vi "Create Table.vi"(6 "CaseSelectInput":bool, 8 "error in (no error)":errorcluster, 9 "ColumnInfo":T2[](array[typedef]), 10 "Table":string, 11 "Refnum in":T1) -> (0 "error out":errorcluster, 3 "Refnum out":T1)   [LabVIEW 2021, in "Database.lvlib"]
uses:
  Database.lvlib
  <vilib>/addons/database/Auxilliary.llb/DB Tools Column Info.ctl
  <vilib>/addons/database/Auxilliary.llb/DB Tools DataTypes.ctl
  <vilib>/addons/database/Connection.llb/Conn ObjectReference.ctl
  <vilib>/addons/database/NI_Database_API.lvlib
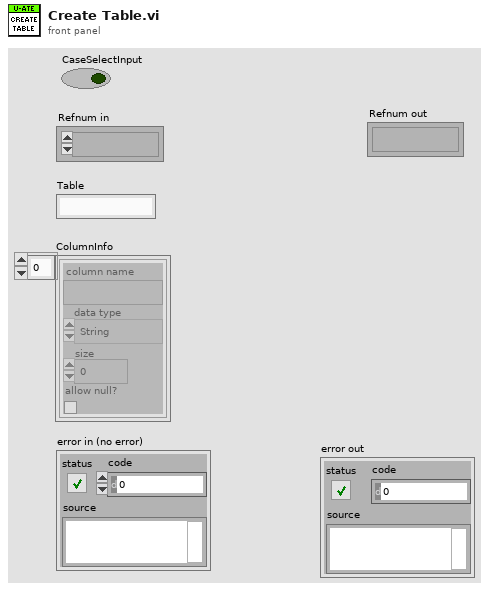
[diagram p1: front panel]
types:
  T1 = typedef "NI_Database_API.lvlib/Conn ObjectReference.ctl" = refnum<k1>
  T2 = typedef "NI_Database_API.lvlib/DB Tools Column Info.ctl" = cluster{"column name":string, "data type":T3, "size":i32, "allow null?":bool}
  T3 = typedef "NI_Database_API.lvlib/DB Tools DataTypes.ctl" = enum16{"String", "Long (I32)", "Single (SGL)", "Double (DBL)", "Date/Time", "Binary"}
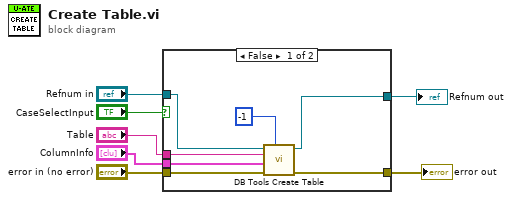
[diagram p0: block diagram]
diagram:
  n1 = case shown="False" "CaseSelectInput" {
    tunnel: "error in (no error)" -> [w13 w15]
    tunnel: "Refnum in" -> [w12 w16]
    tunnel: "Table" -> [w11 _]
    tunnel: "ColumnInfo" -> [w10 _]
    tunnel: [w9 w15] -> w4
    tunnel: [w8 w16] -> w5
    frame False {
      n2 = call <vilib>:"DB Tools Create Table.vi"("primary key (-1)"=-1, "error in (no error)"=w13, "column information"=w10, "table"=w11, "connection reference"=w12) -> ("error out"=w9:errorcluster, "connection reference out"=w8:T1)  [unwired: 3 in]
    }
    frame True {
    }
  }
  "Refnum out" <- w5
  "error out" <- w4
